vi "BME_DG_ResetModuloCounter.vi"(8 "error in (no error)":errorcluster, 11 "DG_Number":i32) -> (0 "error out":errorcluster)   [LabVIEW 2009]
uses:
  BME DLL/DelayGenerator.dll
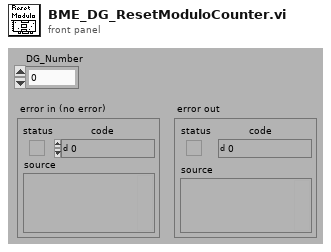
[diagram p1: front panel]
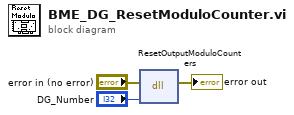
[diagram p0: block diagram]
diagram:
  n1 = dll-call lib="C:/Dokumente und Einstellungen/A2.5/Desktop/POLARIS BME DG/BME DLL/DelayGenerator.dll" fn="ResetOutputModuloCounters" label="Reset Output Modulo Counters"(error in="error in (no error)", "dg_number"="DG_Number") -> (error out=→"error out":errorcluster)  [unwired: 4 in, 1 out]
